vi "XNET.CAN.BusMonitor.Destroy.vi"(8 "error in (no error)":errorcluster, 11 "gRPC Container in":refnum<class "XNET.CAN.BusMonitor.API.lvclass">) -> (0 "error out":errorcluster, 3 "gRPC Container out":refnum<class "XNET.CAN.BusMonitor.API.lvclass">)   [LabVIEW 2025, in "XNET.CAN.BusMonitor.API.lvlib" / "XNET.CAN.BusMonitor.API.lvclass"]
uses:
  XNET.CAN.BusMonitor.API.lvclass
  XNET.CAN.BusMonitor.API.lvclass/XNET.CAN.BusMonitor.API.ctl
  <vilib>/gRPC/LabVIEW gRPC Servicer/ServiceBase/ServiceBase.lvclass
  <vilib>/gRPC/LabVIEW gRPC Servicer/Servicer/Servicer.lvclass
  <vilib>/Utility/SystemLogging/NI_SystemLogging.lvlib
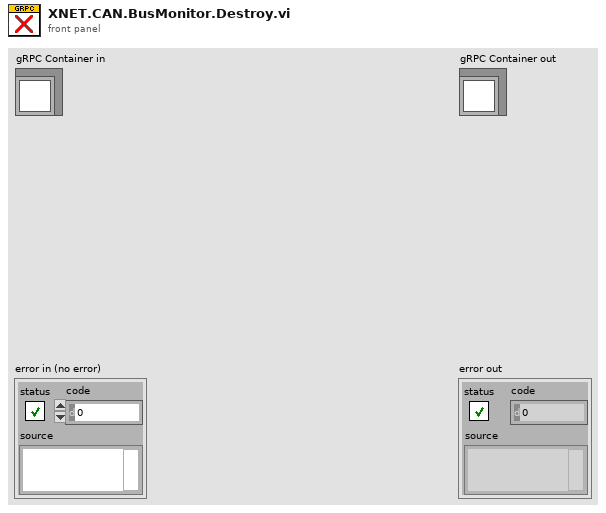
[diagram p1: front panel]
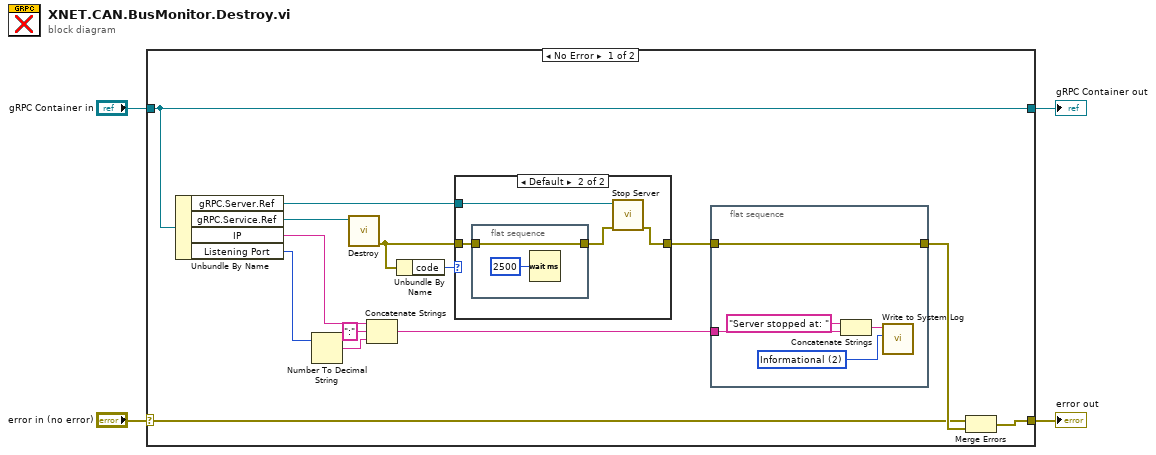
[diagram p0: block diagram]
diagram:
  n1 = case shown="No Error" "error in (no error)" {
    selector: "error in (no error)" -> [w6 w32]
    tunnel: [w5 w32] -> w3
    tunnel: [w16 w31] -> w1
    tunnel: "gRPC Container in" -> [w16 w31]
    frame No Error {
      n2 = Unbundle By Name(w16) -> ("gRPC.Server.Ref"=w14:refnum<class "Servicer.lvclass">, "gRPC.Service.Ref"=w15:refnum<class "ServiceBase.lvclass">, "IP"=w13:string, "Listening Port"=w11:i32)
      n3 = Number To Decimal String(number=w11) -> (decimal integer string=w10:string)  [unwired: 1 in]
      n4 = call-dynamic "Destroy.vi"("gRPC service in"=w15) -> ("error out"=w18:errorcluster)  [unwired: 9 in, 1 out]
      n5 = Concatenate Strings(w13, ":" ("string"), w10) -> (w9:string)
      n6 = Unbundle By Name(w18) -> ("code"=w17:i32)
      n7 = case shown="Default" w17 {
        tunnel: w14 -> [_ w28]
        tunnel: w18 -> [w24 w27]
        tunnel: [w24 w25] -> w8
        frame -8001 {
        }
        frame Default {
          n8 = flat-sequence {
            tunnel: [w29] -> w26
            tunnel: w27 -> [w29]
            frame #0 {
              n9 = Wait (ms)(milliseconds to wait=u32 2500) -> ()  [unwired: 1 out]
            }
          }
          n10 = call <vilib>:"Stop Server.vi"("error in"=w26, "gRPC server in"=w28) -> ("error out"=w25:errorcluster)  [unwired: 9 in]
        }
      }
      n11 = flat-sequence {
        tunnel: w9 -> [w20]
        tunnel: w8 -> [w19]
        tunnel: [w19] -> w7
        frame #0 {
          w22 = 2 items=["Error", "Warning", "Informational"] ("severity")
          n12 = Concatenate Strings("Server stopped at: " ("string"), w20) -> (w21:string)
          n13 = call <vilib>:"Write to System Log.vi"("severity"=w22, "message"=w21) -> ()  [unwired: 9 in, 1 out]
        }
      }
      n14 = Merge Errors(w6, w7) -> (w5:errorcluster)
    }
    frame Error {
    }
  }
  "error out" <- w3
  "gRPC Container out" <- w1
